vi "ryTimer Start Stop.vi"(8 "error in (no error)":errorcluster, 9 "Wait Time ms (0=Use existing)":u32, 10 "Start? (F=Stop)":bool, 11 "Timer in":refnum<class "ryTimer.lvclass">) -> (0 "error out":errorcluster, 3 "Timer out":refnum<class "ryTimer.lvclass">)   [LabVIEW 2021, in "ryTimer.lvclass"]
doc: "Starts or stops the timer. Optionally, set the <b>Wait Time ms</b> to change the time to wait between emits. A value of zero keeps the existing wait time value."
uses:
  ryTimer.lvclass
  ryTimer.lvclass/ryTimer.ctl
  SubVIs/ryTimer Get Properties.vi
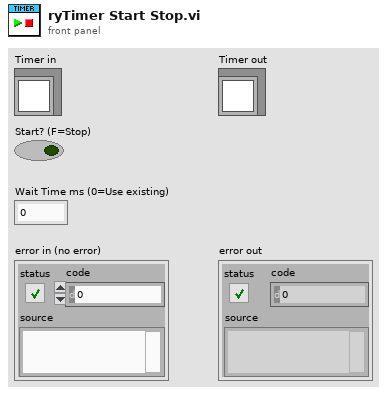
[diagram p1: front panel]
types:
  T1 = typedef "ryTimer.lvclass/ryTimer Properties.ctl" = cluster{"Wait Time (ms)":u32, "Is Running":bool, "Last Sent":u32, "Emit":refnum<queue>}
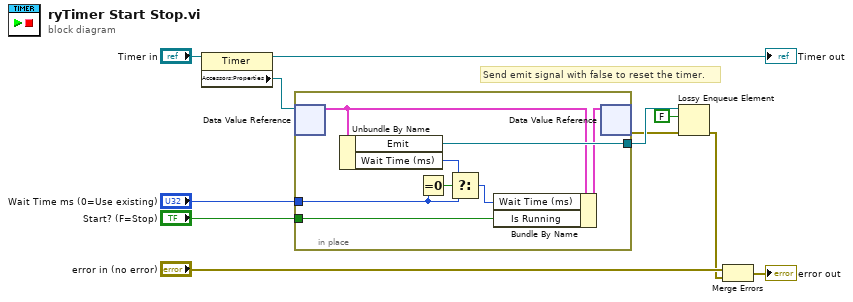
[diagram p0: block diagram]
diagram:
  # "Send emit signal with false to reset the timer."
  n1 = property class="Timer"(reference="Timer in") -> (reference out=→"Timer out":refnum<class "ryTimer.lvclass">, "Accessors:Properties"=w2:refnum<data-value>)  [unwired: 1 in, 1 out]
  n2 = in-place {
    in-place-border: [w19] -> w6
    in-place-border: "Start? (F=Stop)" -> [w18]
    in-place-border: "Wait Time ms (0=Use existing)" -> [w17]
    n3 = in-place-dvr #1(w2) -> (w13:T1)  [unwired: 1 out]
    n4 = Unbundle By Name(w13) -> ("Emit"=w19:refnum<queue>, "Wait Time (ms)"=w15:u32)
    n5 = Equal To 0?(x=w17) -> (x = 0?=w16:bool)
    n6 = Select(t=w15, s=w16, f=w17) -> (s? t:f=w14:u32)
    n7 = Bundle By Name(cluster=w13, "Wait Time (ms)"=w14, "Is Running"=w18) -> (w12:T1)
    n8 = in-place-dvr #1(w12) -> (w1:errorcluster)  [unwired: 1 out]
  }
  n9 = Lossy Enqueue Element(queue=w6, element=FALSE, error in (no error)=w1) -> (error out=w8:errorcluster)  [unwired: 3 out]
  n10 = Merge Errors("error in (no error)", w8) -> (→"error out":errorcluster)
